vi "Write Test Log.vi"(11 "file path (dialog if empty)":path) -> (3 "logfileout":path)   [LabVIEW 2018]
uses:
  Test Parameter Globals_1.0.0.vi
  Test Result File Name Global.vi
  <vilib>/Utility/file.llb/Write Delimited Spreadsheet (string).vi
panel:
  out "error out":errorcluster
  out "date/time string":string
  out "concatenated string":string
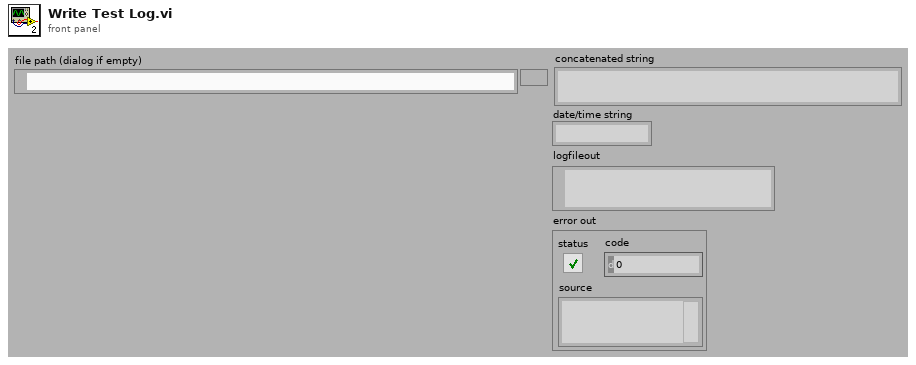
[diagram p1: front panel]
types:
  T1 = enum16{"open", "replace", "create", "open or create", "replace or create", "replace or create with confirmation"}
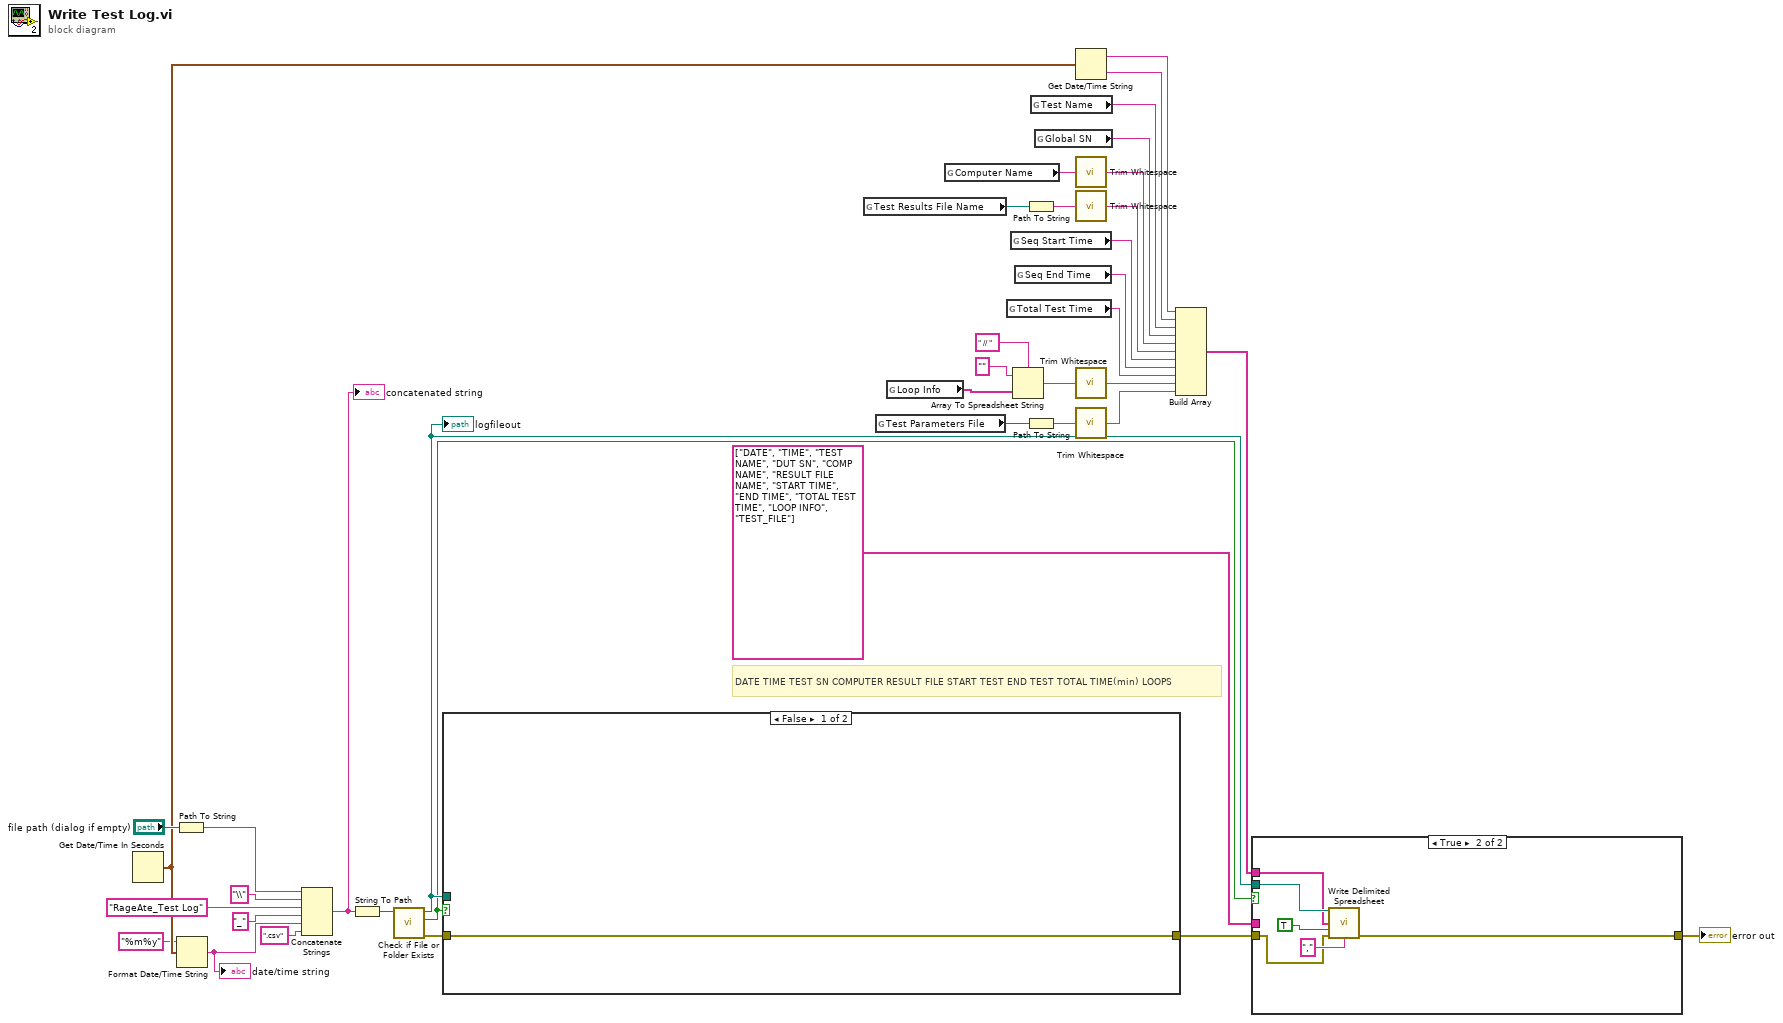
[diagram p0: block diagram]
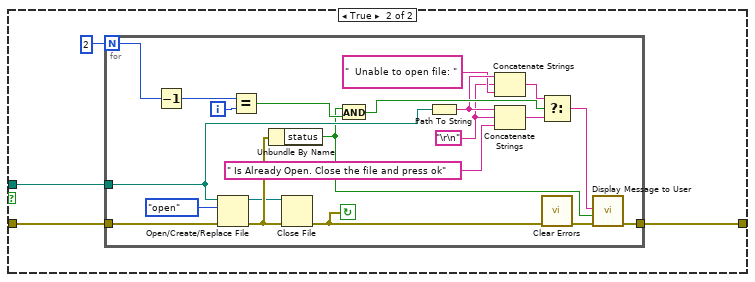
[diagram p2: hidden frame]
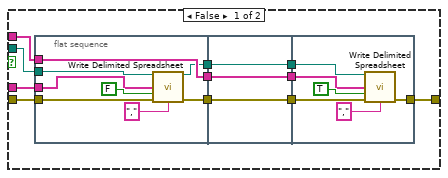
[diagram p3: hidden frame]
diagram:
  # "DATE\tTIME\tTEST\tSN\tCOMPUTER\tRESULT FILE\tSTART TEST\tEND TEST\tTOTAL TIME(min)\tLOOPS"
  n1 = Get Date/Time In Seconds() -> (seconds since 1Jan1904=w18:timestamp)
  n2 = Path To String(path="file path (dialog if empty)") -> (string=w24:string)
  n3 = Format Date/Time String(time format string (%c)="%m%y", seconds (now)=w18) -> (date/time string=w16:string)  [unwired: 1 in]
  "date/time string" <- w16
  n4 = Concatenate Strings(w24, "\\" ("string"), "RageAte_Test Log" ("string"), "_" ("string"), w16, ".csv" ("string")) -> (w15:string)
  "concatenated string" <- w15
  n5 = String To Path(string=w15) -> (path=w14:path)
  n6 = call <vilib>:"Check if File or Folder Exists.vi"("path"=w14) -> ("error out"=w2:errorcluster, "file or folder exists?"=w1:bool, "dup path"=w5:path)  [unwired: 8 in]
  "logfileout" <- w5
  n7 = case shown="False" w1 {
    tunnel: w5 -> [_ w43]
    tunnel: [w39 w41] -> w4
    tunnel: w2 -> [w39 w40]
    frame False {
    }
    frame True {
      n8 = for {
        N: 2 -> [w49]
        tunnel: w43 -> [w63]
        tunnel: [w61] -> w41
        tunnel: w40 -> [w44]
        i -> [w50]
        stop <- w58 continue-if-true
        w45 = "\r\n"
        n9 = Decrement(x=w49) -> (x-1=w48:i32)
        n10 = Open/Create/Replace File(file path (use dialog)=w63, error in=w44, operation (0:open)=T1."open") -> (refnum out=w59:refnum<file>, error out=w60:errorcluster)  [unwired: 3 in, 1 out]
        n11 = Equal?(x=w48, y=w50) -> (x = y?=w57:bool)
        n12 = Unbundle By Name(w60) -> ("status"=w56:bool)
        n13 = Close File(refnum=w59, error in=w60) -> (error out=w58:errorcluster)  [unwired: 1 out]
        n14 = And(x=w56, y=w57) -> (x .and. y?=w54:bool)
        n15 = Path To String(path=w63) -> (string=w53:string)
        n16 = Concatenate Strings(w53, w45, "  Unable to open file: " ("t")) -> (w52:string)
        n17 = Concatenate Strings(w53, w45, " Is Already Open. Close the file and press ok" ("string")) -> (w55:string)
        n18 = Select(t=w52, s=w54, f=w55) -> (s? t:f=w51:string)
        n19 = call <vilib>:"Clear Errors.vi"("error in (no error)"=w58) -> ("error out"=w62:errorcluster)  [unwired: 5 in, 1 out]
        n20 = call "Display Message to User"("error in (no error)"=w62, "Enable"=w56, "Message"=w51) -> ("error out"=w61:errorcluster)  [unwired: 7 in, 1 out]
      }
    }
  }
  n21 = global read "Test Result File Name Global.vi" "Test Results File Name"() -> (w38:path)
  n22 = global read "Test Parameter Globals_1.0.0.vi" "Test Parameters File"() -> (w9:path)
  n23 = global read "Test Parameter Globals_1.0.0.vi" "Loop Info"() -> (w29:string[])
  n24 = global read "Test Parameter Globals_1.0.0.vi" "Computer Name"() -> (w34:string)
  n25 = global read "Test Parameter Globals_1.0.0.vi" "Total Test Time"() -> (w30:string)
  n26 = global read "Test Parameter Globals_1.0.0.vi" "Seq Start Time"() -> (w32:string)
  n27 = Array To Spreadsheet String(delimiter (Tab)=" // ", array=w29, 3:"" ("format string")) -> (spreadsheet string=w26:string)
  n28 = global read "Test Parameter Globals_1.0.0.vi" "Seq End Time"() -> (w31:string)
  n29 = Path To String(path=w38) -> (string=w33:string)
  n30 = Path To String(path=w9) -> (string=w8:string)
  n31 = global read "Test Parameter Globals_1.0.0.vi" "Test Name"() -> (w36:string)
  n32 = global read "Test Parameter Globals_1.0.0.vi" "Global SN"() -> (w35:string)
  n33 = Get Date/Time String(seconds (now)=w18) -> (date string=w19:string, time string=w37:string)  [unwired: 2 in]
  n34 = call <vilib>:"Trim Whitespace.vi"("string"=w34) -> ("trimmed string"=w10:string)  [unwired: 1 in]
  n35 = call <vilib>:"Trim Whitespace.vi"("string"=w33) -> ("trimmed string"=w11:string)  [unwired: 1 in]
  n36 = call <vilib>:"Trim Whitespace.vi"("string"=w26) -> ("trimmed string"=w6:string)  [unwired: 1 in]
  n37 = call <vilib>:"Trim Whitespace.vi"("string"=w8) -> ("trimmed string"=w7:string)  [unwired: 1 in]
  n38 = Build Array(w19, w37, w36, w35, w10, w11, w32, w31, w30, w6, w7) -> (w13:string[])
  n39 = case shown="True" w1 {
    tunnel: w5 -> [w75 w96]
    tunnel: w13 -> [w72 w95]
    tunnel: string[] ["DATE", "TIME", "TEST NAME", "DUT SN", "COMP NAME", "RESULT FILE NAME", "START TIME", "END TIME", "TOTAL TEST TIME", "LOOP INFO", "TEST_FILE"] -> [w69 _]
    tunnel: w4 -> [w68 w94]
    tunnel: [w65 w93] -> w3
    frame False {
      n40 = flat-sequence {
        tunnel: w75 -> [w82]
        tunnel: [w80] -> w73
        tunnel: w72 -> [w80]
        tunnel: [w79] -> w70
        tunnel: w69 -> [w78]
        tunnel: w68 -> [w77]
        tunnel: [w76] -> w67
        tunnel: [w86] -> w74
        tunnel: w73 -> [w86]
        tunnel: [w85] -> w71
        tunnel: w70 -> [w85]
        tunnel: w67 -> [w84]
        tunnel: [w84] -> w66
        tunnel: w74 -> [w89]
        tunnel: w71 -> [w92]
        tunnel: w66 -> [w88]
        tunnel: [w87] -> w65
        frame #0 {
          n41 = call-poly <vilib>:"Write Delimited Spreadsheet.vi"("file path (dialog if empty)"=w82, "1D data"=w78, "append to file? (new file:F)"=FALSE, "error in (no error)"=w77, "delimiter (\\t)"="," ("delimiter (\\t)")) -> ("new file path (Not A Path if cancelled)"=w79:path, "error out"=w76:errorcluster)  [unwired: 9 in]
        }
        frame #1 {
        }
        frame #2 {
          n42 = call-poly <vilib>:"Write Delimited Spreadsheet.vi"("file path (dialog if empty)"=w92, "1D data"=w89, "append to file? (new file:F)"=TRUE, "error in (no error)"=w88, "delimiter (\\t)"="," ("delimiter (\\t)")) -> ("error out"=w87:errorcluster)  [unwired: 9 in, 1 out]
        }
      }
    }
    frame True {
      n43 = call-poly <vilib>:"Write Delimited Spreadsheet.vi"("file path (dialog if empty)"=w96, "1D data"=w95, "append to file? (new file:F)"=TRUE, "error in (no error)"=w94, "delimiter (\\t)"="," ("delimiter (\\t)")) -> ("error out"=w93:errorcluster)  [unwired: 9 in, 1 out]
    }
  }
  "error out" <- w3
